vi "initiate.vi"(8 "error in (no error)":errorcluster, 11 "reference in":refnum<class "File Controller.lvclass">) -> (0 "error out":errorcluster, 3 "reference out":refnum<class "File Controller.lvclass">)   [LabVIEW 2015, in "File Controller.lvclass"]
uses:
  File Controller.lvclass
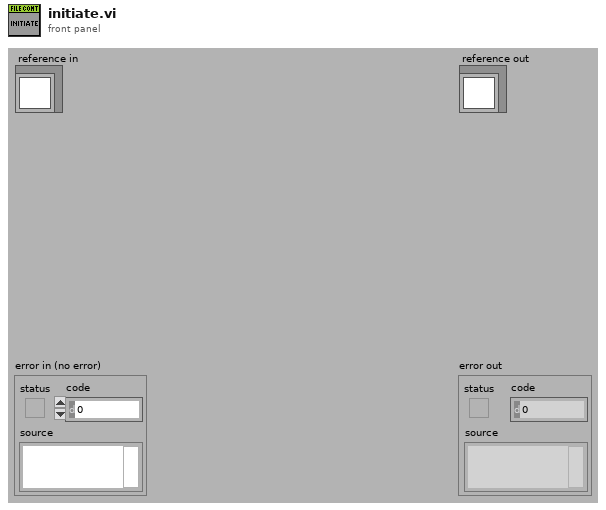
[diagram p1: front panel]
types:
  T1 = typedef "File Controller.lvclass/ObjectAttributesRef.ctl" = refnum<data-value>
  T2 = typedef "File Controller.lvclass/ObjectAttributes.ctl" = cluster{"MyAttribute":dbl, "file_path":path, "file_type":T3, "data":string[][][], "excel_file_ref":refnum<class "excelFile.lvclass">, "sheetName":string[], "subject_refs":refnum<class "subject.lvclass">[], "temp_data":string[][][]}
  T3 = typedef "excelFile.lvclass/fileType.ctl" = enum16{"database", "CosmedTest"}
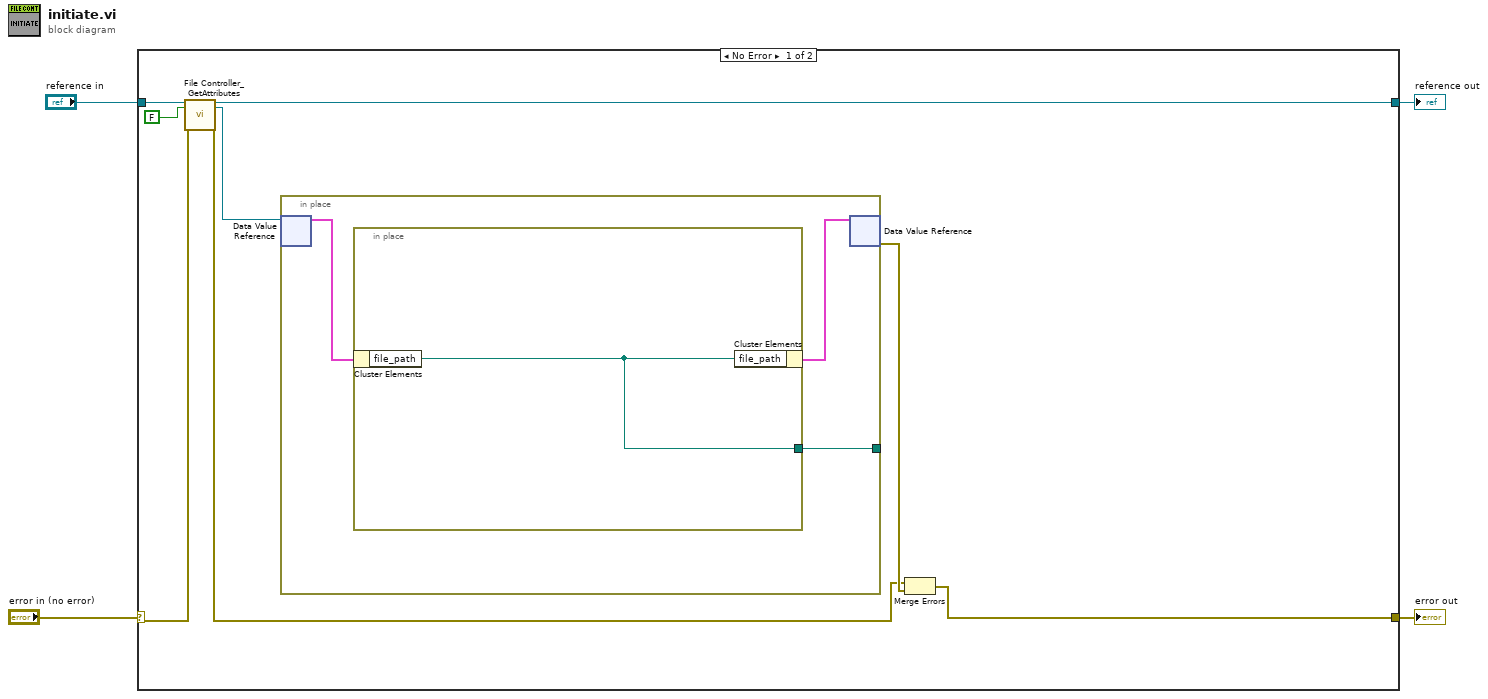
[diagram p0: block diagram]
diagram:
  n1 = case shown="No Error" "error in (no error)" {
    selector: "error in (no error)" -> [w10 w17]
    tunnel: [w6 w18] -> w2
    tunnel: "reference in" -> [w12 w18]
    tunnel: [w5 w17] -> w1
    frame No Error {
      n2 = call "File Controller_GetAttributes.vi"("reference in"=w12, "return data? (T)"=FALSE, "error in (no error)"=w10) -> ("reference out"=w6:refnum<class "File Controller.lvclass">, "attributes ref"=w9:T1, "error out"=w7:errorcluster)  [unwired: 13 in, 1 out]
      n3 = in-place {
        in-place-border: [w13] -> _
        n4 = in-place-dvr #1(w9) -> (w14:T2)  [unwired: 1 out]
        n5 = in-place {
          in-place-border: [w16] -> w13
          n6 = in-place-cluster #2(w14) -> ("file_path"=w16:path)
          n7 = in-place-cluster #2("file_path"=w16) -> (w15:T2)
        }
        n8 = in-place-dvr #1(w15) -> (w8:errorcluster)  [unwired: 1 out]
      }
      n9 = Merge Errors(w7, w8) -> (w5:errorcluster)
    }
    frame Error {
    }
  }
  "error out" <- w1
  "reference out" <- w2
